vi "MGCC_MdlMgmt_Data-write-to-txt.vi"   [LabVIEW 2016]
doc: "-----------------------------------------------------------------------------------------------------------------------\nCopyright <2019> <The University of Tennessee at Knoxville and the University of Tennessee Research Foundation>\nThis software is released under BSD-3 \nhttps://opensource.org/licenses/BSD-3-Clause \nAdditional license options available at https://utrf.tennessee.edu/industry/sample-agreements/\n-----------------------------------------------------------------------------------------------------------------------"
types:
  T1 = enum16{"open", "replace", "create", "open or create", "replace or create", "replace or create with confirmation"}
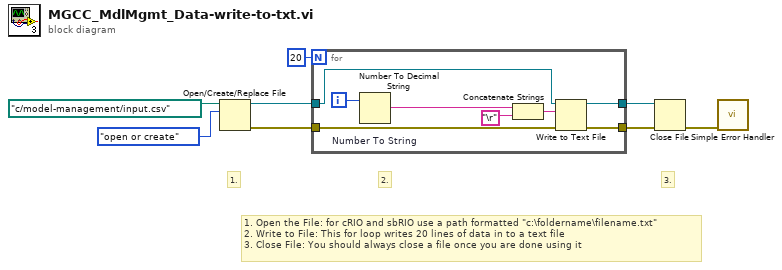
[diagram p0: block diagram]
diagram:
  # "1. Open the File: for cRIO and sbRIO use a path formatted \"c:\\foldername\\filename.txt\"\n2. Write to File: This for loop writes 20 lines of data in to a text file\n3. Close File: You should always close a file once you are done using it"
  # "3."
  # "2."
  # "1."
  n1 = Open/Create/Replace File(file path (use dialog)=path "c:/model-management/input.csv", operation (0:open)=T1."open or create") -> (refnum out=w8:refnum<file>, error out=w6:errorcluster)  [unwired: 4 in, 1 out]
  n2 = for {
    N: 20 -> [_]
    tunnel: [w16] -> w2
    tunnel: w8 -> [w15]
    tunnel: w6 -> [w14]
    tunnel: [w13] -> w1
    i -> [w12]
    n3 = Number To Decimal String "Number To String"(number=w12) -> (decimal integer string=w11:string)  [unwired: 1 in]
    n4 = Concatenate Strings(w11, "\r") -> (w9:string)
    n5 = Write to Text File(file (use dialog)=w15, text=w9, error in=w14) -> (refnum out=w16:refnum<file>, error out=w13:errorcluster)  [unwired: 1 in, 1 out]
  }
  n6 = Close File(refnum=w2, error in=w1) -> (error out=w4:errorcluster)  [unwired: 1 out]
  n7 = call <vilib>:"Simple Error Handler.vi"("error in (no error)"=w4) -> ()  [unwired: 4 in, 5 out]
